vi "Pianino.vi"() -> ()   [LabVIEW 2018]
uses:
  <vilib>/sound2/lvsound2.llb/Sound Data Format.ctl
  <vilib>/sound2/lvsound2.llb/Sampling Mode.ctl
  <vilib>/Utility/inputDevices.llb/keyboardAcquire.vi
  <vilib>/sound2/lvsound2.llb/Sound Output Set Volume (Single).vi
  <vilib>/Utility/inputDevices.llb/closeKeyboard.vi
  <vilib>/sound2/lvsound2.llb/Sound Output Write (DBL Single).vi
  <vilib>/measure/NI_MABase.lvlib
panel:
  in  "Oktawa":dbl
  out "B":bool
  out "A":bool
  out "G":bool
  out "F":bool
  out "E":bool
  out "D":bool
  out "C":bool
  in  "?":bool
  # "2 - wielka \n1 - mała\n0 - razkreślna\n-1 -dwukreślna\n-2 - trzykreślna"
  # "STOP"
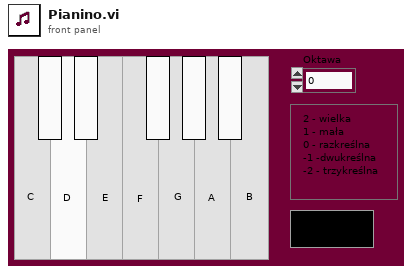
[diagram p1: front panel]
types:
  T1 = typedef "Sampling Mode.ctl" = i32
  T2 = typedef "Sound Data Format.ctl" = cluster{"sample rate (S/s)":dbl, "number of channels":i32, "bits per sample":i32}
  T3 = typedef "Sound Output Task ID.ctl" = u32
  T4 = enum16{"0", "1", "2", "3", "4", "5", "6", "7", "8", "9", "A", "B", "C", "D", "E", "F", "G", "H", "I", "J", "K", "L", "M", "N", "O", "P", "Q", "R", "S", "T", "U", "V", "W", "X", "Y", "Z", "F1", "F2", "F3", "F4", "F5", "F6", "F7", "F8", "F9", "F10", "F11", "F12", "F13", "F14", "F15", "ADD", "BACK", "BACKSLASH", "CAPITAL", "COMMA", "DECIMAL", "DELETE", "DIVIDE", "DOWN", "END", "EQUALS", "ESCAPE", "GRAVE (`)", "HOME", "INSERT", "LBRACKET", "LCONTROL", "LEFT", "L ALT", "LSHIFT", "LWIN", "MINUS", "MULTIPLY", "NEXT", "NUMLOCK", "NUMPAD_0", "NUMPAD_1", "NUMPAD_2", "NUMPAD_3", "NUMPAD_4", "NUMPAD_5", "NUMPAD_6", "NUMPAD_7", "NUMPAD_8", "NUMPAD_9", "PAUSE", "PERIOD", "PRIOR (PG UP)", "RBRACKET", "RCONTROL", "RETURN", "RIGHT", "R ALT", "RSHIFT", "RWIN", "SCROLL", "SEMICOLON", "SLASH", "SPACE", "SUBTRACT", "TAB", "UP", "ENTER (num pad)", "' (quote)"}[]
  T5 = enum16{"0", "1", "2", "3", "4", "5", "6", "7", "8", "9", "A", "B", "C", "D", "E", "F", "G", "H", "I", "J", "K", "L", "M", "N", "O", "P", "Q", "R", "S", "T", "U", "V", "W", "X", "Y", "Z", "F1", "F2", "F3", "F4", "F5", "F6", "F7", "F8", "F9", "F10", "F11", "F12", "F13", "F14", "F15", "ADD", "BACK", "BACKSLASH", "CAPITAL", "COMMA", "DECIMAL", "DELETE", "DIVIDE", "DOWN", "END", "EQUALS", "ESCAPE", "GRAVE (`)", "HOME", "INSERT", "LBRACKET", "LCONTROL", "LEFT", "L ALT", "LSHIFT", "LWIN", "MINUS", "MULTIPLY", "NEXT", "NUMLOCK", "NUMPAD_0", "NUMPAD_1", "NUMPAD_2", "NUMPAD_3", "NUMPAD_4", "NUMPAD_5", "NUMPAD_6", "NUMPAD_7", "NUMPAD_8", "NUMPAD_9", "PAUSE", "PERIOD", "PRIOR (PG UP)", "RBRACKET", "RCONTROL", "RETURN", "RIGHT", "R ALT", "RSHIFT", "RWIN", "SCROLL", "SEMICOLON", "SLASH", "SPACE", "SUBTRACT", "TAB", "UP", "ENTER (num pad)", "' (quote)"}
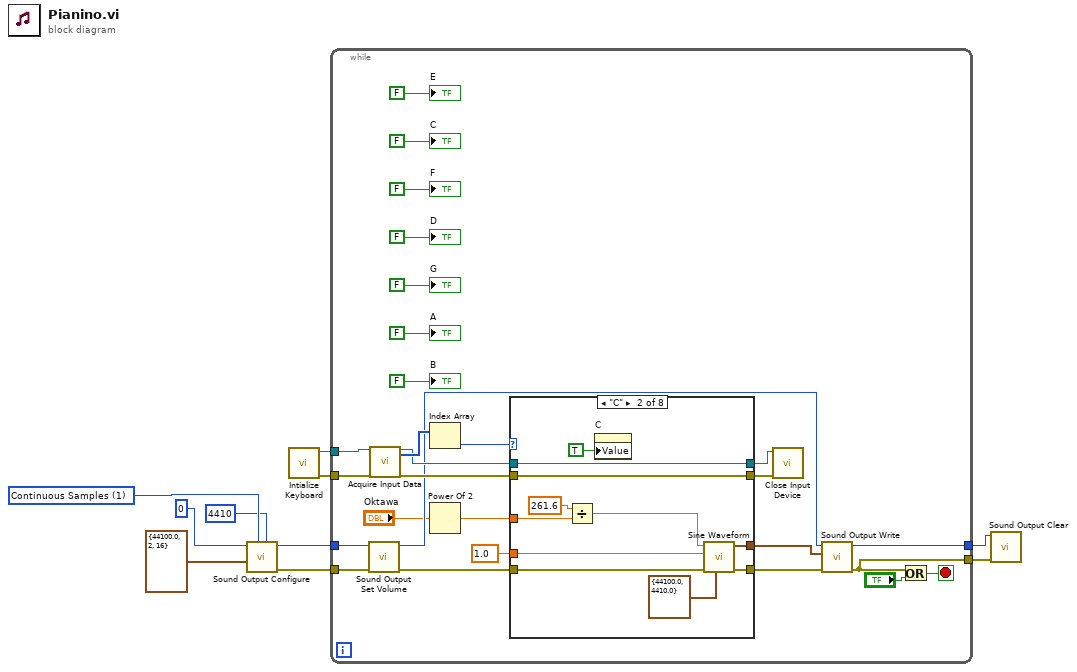
[diagram p0: block diagram]
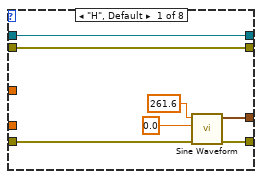
[diagram p2: hidden frame]
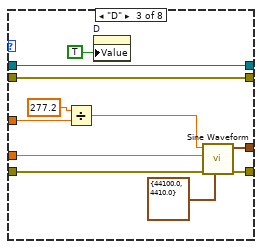
[diagram p3: hidden frame]
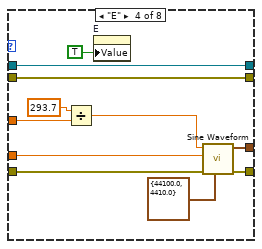
[diagram p4: hidden frame]
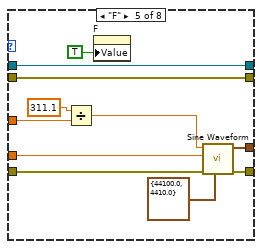
[diagram p5: hidden frame]
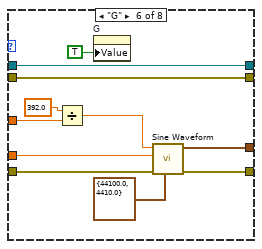
[diagram p6: hidden frame]
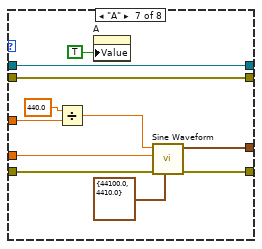
[diagram p7: hidden frame]
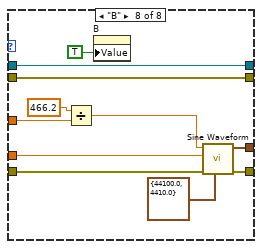
[diagram p8: hidden frame]
diagram:
  w8 = T1 1 items=["Finite Samples", "Continuous Samples"] ("sample mode")
  n1 = call <vilib>:"Sound Output Configure.vi"("number of samples/ch"=4410, "sample mode"=w8, "sound format"=T2 {"sample rate (S/s)"=44100.0, "number of channels"=2, "bits per sample"=16}, "device ID"=u32 0) -> ("error out"=w5:errorcluster, "task ID"=w6:T3)  [unwired: 6 in]
  n2 = call <vilib>:"Intialize Keyboard.vi"() -> ("error out"=w3:errorcluster, "device ID"=w4:refnum<k1>)  [unwired: 10 in]
  n3 = while {
    tunnel: w6 -> [w38]
    tunnel: w5 -> [w37]
    tunnel: w4 -> [w34]
    tunnel: w3 -> [w33]
    tunnel: [w22] -> w2
    tunnel: [w21] -> w1
    stop <- w35 stop-if-true
    n4 = call-poly <vilib>:"Sound Output Set Volume.vi"("error in (no error)"=w37, "task ID"=w38) -> ("error out"=w28:errorcluster, "task ID out"=w23:T3)  [unwired: 8 in]
    n5 = call-poly <vilib>:"Acquire Input Data.vi"("device ID"=w34, "error in (no error)"=w33) -> ("device ID"=w25:refnum<k1>, "keys pressed"=w32:T4, "error out"=w26:errorcluster)  [unwired: 15 in]
    n6 = Index Array(array=w32) -> (element=w31:T5)  [unwired: 1 in]
    n7 = Power Of 2(x="Oktawa") -> (2^x=w12:dbl)
    n8 = case shown="\"C\"" w31 {
      tunnel: [w41 w56 w63 w74 w85 w94 w107 w118] -> w29
      tunnel: [w42 w55 w64 w75 w86 w96 w108 w119] -> w30
      tunnel: w28 -> [w43 w54 w65 w76 w87 w97 w109 w120]
      tunnel: 1.0 ("amplitude") -> [_ w53 w66 w77 w88 w95 w110 w121]
      tunnel: w26 -> [w39 w52 w61 w72 w83 w98 w105 w116]
      tunnel: w25 -> [w40 w51 w62 w73 w84 w99 w106 w117]
      tunnel: [w40 w51 w62 w73 w84 w99 w106 w117] -> w24
      tunnel: [w39 w52 w61 w72 w83 w98 w105 w116] -> w20
      tunnel: w12 -> [_ w47 w57 w69 w80 w91 w101 w114]
      frame "H", Default {
        n9 = call <vilib>:"Sine Waveform.vi"("error in (no error)"=w43, "amplitude"=0.0, "frequency"=261.6) -> ("error out"=w42:errorcluster, "signal out"=w41:waveform(dbl))  [unwired: 7 in]
      }
      frame "C" {
        n10 = Divide(x=261.6 ("frequency"), y=w47) -> (x/y=w48:dbl)
        n11 = property on="C" class="Bool (strict)"("Value"=TRUE) -> ()  [unwired: 2 in, 2 out]
        n12 = call <vilib>:"Sine Waveform.vi"("sampling info"=cluster{"Fs":dbl, "#s":dbl} {"Fs"=44100.0, "#s"=4410.0}, "error in (no error)"=w54, "amplitude"=w53, "frequency"=w48) -> ("error out"=w55:errorcluster, "signal out"=w56:waveform(dbl))  [unwired: 6 in]
      }
      frame "D" {
        n13 = Divide(x=277.2 ("frequency"), y=w57) -> (x/y=w58:dbl)
        n14 = property on="D" class="Bool (strict)"("Value"=TRUE ("D")) -> ()  [unwired: 2 in, 2 out]
        n15 = call <vilib>:"Sine Waveform.vi"("sampling info"=cluster{"Fs":dbl, "#s":dbl} {"Fs"=44100.0, "#s"=4410.0}, "error in (no error)"=w65, "amplitude"=w66, "frequency"=w58) -> ("error out"=w64:errorcluster, "signal out"=w63:waveform(dbl))  [unwired: 6 in]
      }
      frame "E" {
        n16 = Divide(x=293.7 ("frequency"), y=w69) -> (x/y=w68:dbl)
        n17 = property on="E" class="Bool (strict)"("Value"=TRUE ("E")) -> ()  [unwired: 2 in, 2 out]
        n18 = call <vilib>:"Sine Waveform.vi"("sampling info"=cluster{"Fs":dbl, "#s":dbl} {"Fs"=44100.0, "#s"=4410.0}, "error in (no error)"=w76, "amplitude"=w77, "frequency"=w68) -> ("error out"=w75:errorcluster, "signal out"=w74:waveform(dbl))  [unwired: 6 in]
      }
      frame "F" {
        n19 = Divide(x=311.1 ("frequency"), y=w80) -> (x/y=w79:dbl)
        n20 = property on="F" class="Bool (strict)"("Value"=TRUE ("F")) -> ()  [unwired: 2 in, 2 out]
        n21 = call <vilib>:"Sine Waveform.vi"("sampling info"=cluster{"Fs":dbl, "#s":dbl} {"Fs"=44100.0, "#s"=4410.0}, "error in (no error)"=w87, "amplitude"=w88, "frequency"=w79) -> ("error out"=w86:errorcluster, "signal out"=w85:waveform(dbl))  [unwired: 6 in]
      }
      frame "G" {
        n22 = Divide(x=392.0 ("frequency"), y=w91) -> (x/y=w90:dbl)
        n23 = property on="G" class="Bool (strict)"("Value"=TRUE ("G")) -> ()  [unwired: 2 in, 2 out]
        n24 = call <vilib>:"Sine Waveform.vi"("sampling info"=cluster{"Fs":dbl, "#s":dbl} {"Fs"=44100.0, "#s"=4410.0}, "error in (no error)"=w97, "amplitude"=w95, "frequency"=w90) -> ("error out"=w96:errorcluster, "signal out"=w94:waveform(dbl))  [unwired: 6 in]
      }
      frame "A" {
        n25 = Divide(x=440.0 ("frequency"), y=w101) -> (x/y=w102:dbl)
        n26 = property on="A" class="Bool (strict)"("Value"=TRUE ("A")) -> ()  [unwired: 2 in, 2 out]
        n27 = call <vilib>:"Sine Waveform.vi"("sampling info"=cluster{"Fs":dbl, "#s":dbl} {"Fs"=44100.0, "#s"=4410.0}, "error in (no error)"=w109, "amplitude"=w110, "frequency"=w102) -> ("error out"=w108:errorcluster, "signal out"=w107:waveform(dbl))  [unwired: 6 in]
      }
      frame "B" {
        n28 = Divide(x=466.2 ("frequency"), y=w114) -> (x/y=w112:dbl)
        n29 = property on="B" class="Bool (strict)"("Value"=TRUE ("B")) -> ()  [unwired: 2 in, 2 out]
        n30 = call <vilib>:"Sine Waveform.vi"("sampling info"=cluster{"Fs":dbl, "#s":dbl} {"Fs"=44100.0, "#s"=4410.0}, "error in (no error)"=w120, "amplitude"=w121, "frequency"=w112) -> ("error out"=w119:errorcluster, "signal out"=w118:waveform(dbl))  [unwired: 6 in]
      }
    }
    n31 = call-poly <vilib>:"Close Input Device.vi"("error in (no error)"=w20, "device ID"=w24) -> ()  [unwired: 8 in, 1 out]
    n32 = call-poly <vilib>:"Sound Output Write.vi"("error in (no error)"=w30, "data"=w29, "task ID"=w23) -> ("error out"=w22:errorcluster, "task ID out"=w21:T3)  [unwired: 7 in]
    n33 = Or(x=w22, y="?") -> (x .or. y?=w35:bool)
    "C" <- FALSE ("C")
    "D" <- FALSE ("D")
    "E" <- FALSE ("E")
    "F" <- FALSE ("F")
    "G" <- FALSE ("G")
    "A" <- FALSE ("A")
    "B" <- FALSE ("B")
  }
  n34 = call <vilib>:"Sound Output Clear.vi"("error in (no error)"=w2, "task ID"=w1) -> ()  [unwired: 9 in, 1 out]
